vi "Teleop.vi"(10 "Match Info":T1={"Autonomous Elapsed Seconds"=0.0, "TeleOp Elapsed Seconds"=0.0, "Disabled Elapsed Seconds"=0.0, "Visited Autonomous"=FALSE, "Visited TeleOp"=FALSE, "Visited Disabled"=FALSE, "Autonomous Settings"={"Autonomous Style"=enum."Independent", "VI Refnum"=refnum}}, 11 "Call Context":T2) -> ()   [LabVIEW 2013]
doc: "This VI is called for each TeleOp packet received from the DS where the robot is not disabled. It is often used to read from the joysticks and update I/O or to update setpoints for timed control loops. It should complete and return within 20 milliseconds or it may miss DS packets."
uses:
  <vilib>/Rock Robotics/WPI/DriverStation/WPI_DriverStationDerivedRobotMode.ctl
  <vilib>/Rock Robotics/WPI/DriverStation/WPI_DriverStationMatch Info.ctl
  Robot Global Data.vi
  <vilib>/Rock Robotics/WPI/Joystick/WPI_JoystickGetSetRefNum.vi
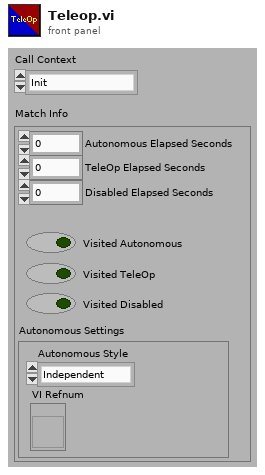
[diagram p1: front panel]
types:
  T1 = typedef "WPI_DriverStationMatch Info.ctl" = cluster{"Autonomous Elapsed Seconds":dbl, "TeleOp Elapsed Seconds":dbl, "Disabled Elapsed Seconds":dbl, "Visited Autonomous":bool, "Visited TeleOp":bool, "Visited Disabled":bool, "Autonomous Settings":cluster{"Autonomous Style":enum16{"Iterative", "Independent"}, "VI Refnum":refnum<vi>}}
  T2 = typedef "WPI_DriverStationDerivedRobotMode.ctl" = enum16{"Init", "Execute", "Stop"}
  T3 = typedef "WPI_JoystickDevRef.ctl" = cluster{"Device":T4}
  T4 = typedef "WPI_JoystickDeviceEnum.ctl" = enum16{"USB 1", "USB 2", "USB 3", "USB 4", "Kinect 1", "Kinect 2"}
  T5 = typedef "WPI_JoystickButtonState.ctl" = cluster{"Button 1":bool, "Button 2":bool, "Button 3":bool, "Button 4":bool, "Button 5":bool, "Button 6":bool, "Button 7":bool, "Button 8":bool, "Button 9":bool, "Button 10":bool, "Button 11":bool, "Button 12":bool}
  T6 = cluster{"axis 1 (x)":dbl, "axis 2 (y)":dbl, "axis 3 (throttle)":dbl, "axis 4":dbl, "axis 5":dbl, "axis 6":dbl}
  T7 = cluster{"X-Axis":dbl, "Y-Axis":dbl, "Bottom Lever":dbl, "Trigger":bool, "Button 2":bool, "Button 3":bool, "Button 4":bool, "Button 5":bool, "Button 6":bool, "Button 7":bool, "Button 8":bool, "Button 9":bool, "Button 10":bool, "Button 11":bool}
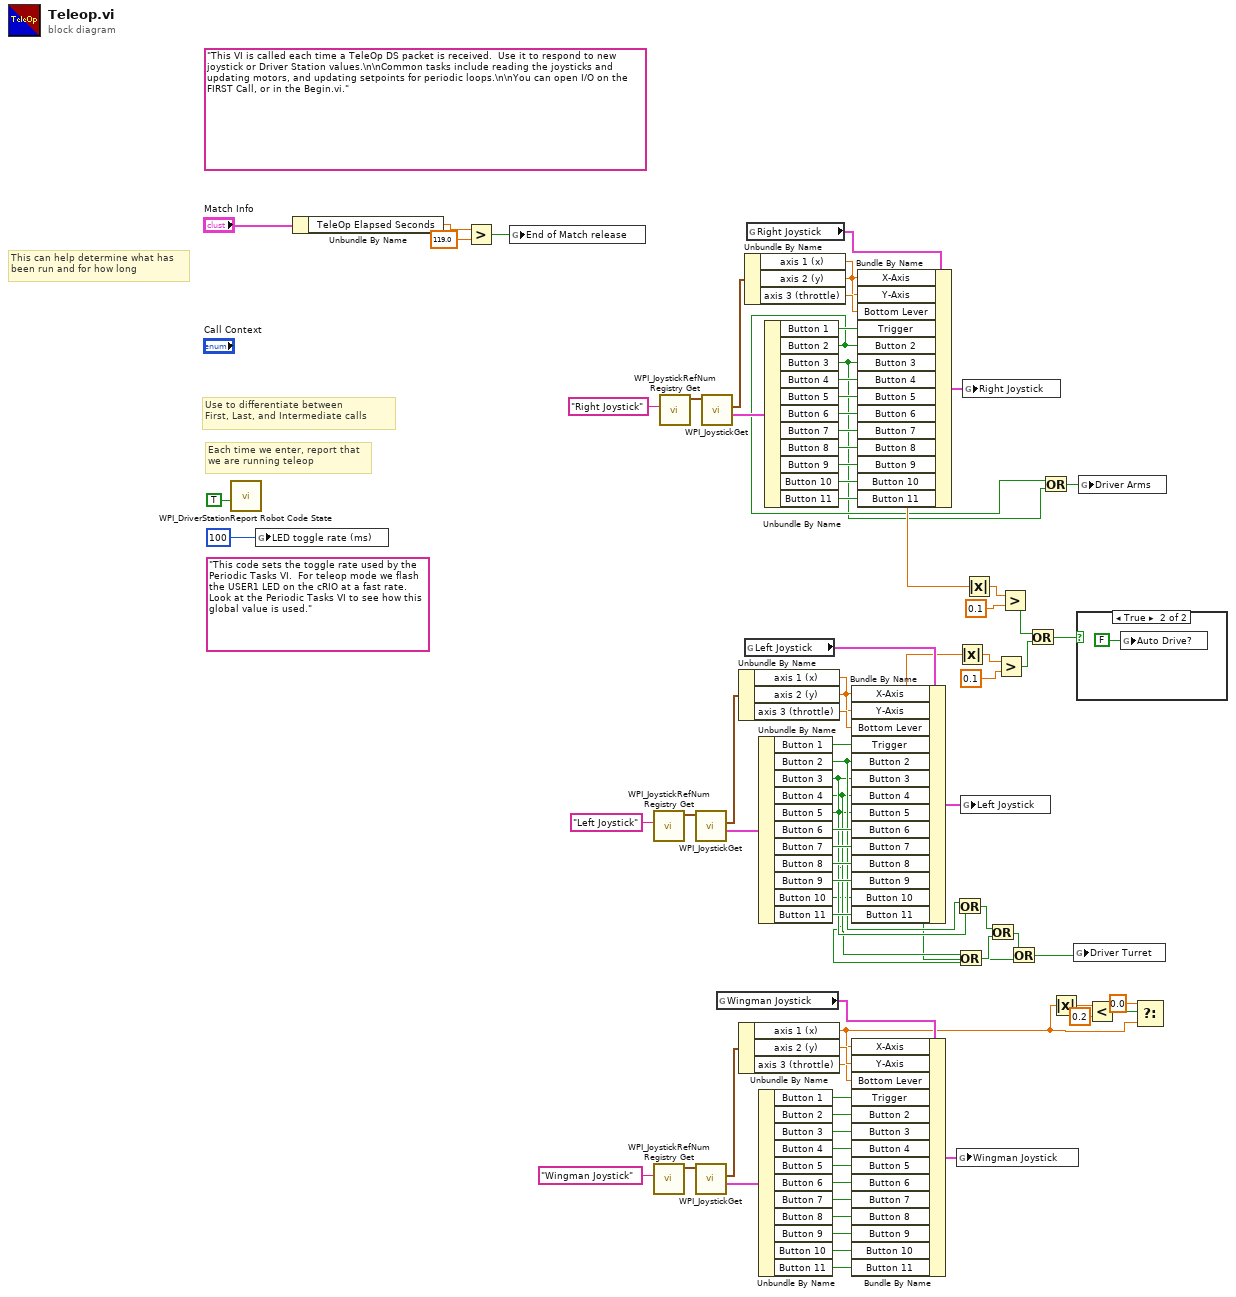
[diagram p0: block diagram]
diagram:
  (unwired) "This code sets the toggle rate used by the Periodic Tasks VI.  For teleop mode we flash the USER1 LED on the cRIO at a fast rate.  Look at the Periodic Tasks VI to see how this global value is used."
  (unwired) "This VI is called each time a TeleOp DS packet is received.  Use it to respond to new joystick or Driver Station values.\n\nCommon tasks include reading the joysticks and updating motors, and updating setpoints for periodic loops.\n\nYou can open I/O on the FIRST Call, or in the Begin.vi."
  # "Each time we enter, report that\nwe are running teleop"
  # "Use to differentiate between\nFirst, Last, and Intermediate calls"
  # "This can help determine what has\nbeen run and for how long"
  n1 = call <vilib>:"WPI_DriverStationReport Robot Code State.vi"("TeleOp"=TRUE ("Autonomous")) -> ()  [unwired: 10 in, 1 out]
  n2 = global write "Robot Global Data.vi" "LED toggle rate (ms)"(u32 100 ("LED ms toggle rate")) -> ()
  n3 = Unbundle By Name("Match Info") -> ("TeleOp Elapsed Seconds"=w39:dbl)
  n4 = Greater?(x=w39, y=119.0) -> (0:w37:bool)
  n5 = global write "Robot Global Data.vi" "End of Match release"(w37) -> ()
  n6 = call <vilib>:"WPI_JoystickRefNum Registry Get.vi"("refnum name"="Left Joystick") -> ("JoystickDevRef"=w61:T3)  [unwired: 9 in, 1 out]
  n7 = call <vilib>:"WPI_JoystickRefNum Registry Get.vi"("refnum name"="Wingman Joystick") -> ("JoystickDevRef"=w35:T3)  [unwired: 9 in, 1 out]
  n8 = call <vilib>:"WPI_JoystickRefNum Registry Get.vi"("refnum name"="Right Joystick") -> ("JoystickDevRef"=w78:T3)  [unwired: 9 in, 1 out]
  n9 = call <vilib>:"WPI_JoystickGet.vi"("JoystickDevRef"=w61) -> ("Buttons"=w59:T5, "Axes"=w60:T6)  [unwired: 4 in, 1 out]
  n10 = call <vilib>:"WPI_JoystickGet.vi"("JoystickDevRef"=w35) -> ("Buttons"=w33:T5, "Axes"=w34:T6)  [unwired: 4 in, 1 out]
  n11 = call <vilib>:"WPI_JoystickGet.vi"("JoystickDevRef"=w78) -> ("Buttons"=w76:T5, "Axes"=w77:T6)  [unwired: 4 in, 1 out]
  n12 = global read "Robot Global Data.vi" "Wingman Joystick"() -> (w32:T7)
  n13 = Unbundle By Name(w60) -> ("axis 1 (x)"=w58:dbl, "axis 2 (y)"=w48:dbl, "axis 3 (throttle)"=w57:dbl)
  n14 = Unbundle By Name(w34) -> ("axis 1 (x)"=w4:dbl, "axis 2 (y)"=w30:dbl, "axis 3 (throttle)"=w29:dbl)
  n15 = Unbundle By Name(w77) -> ("axis 1 (x)"=w73:dbl, "axis 2 (y)"=w47:dbl, "axis 3 (throttle)"=w72:dbl)
  n16 = global read "Robot Global Data.vi" "Left Joystick"() -> (w50:T7)
  n17 = global read "Robot Global Data.vi" "Right Joystick"() -> (w75:T7)
  n18 = Unbundle By Name(w59) -> ("Button 1"=w56:bool, "Button 2"=w17:bool, "Button 3"=w16:bool, "Button 4"=w15:bool, "Button 5"=w14:bool, "Button 6"=w55:bool, "Button 7"=w54:bool, "Button 8"=w53:bool, "Button 9"=w52:bool, "Button 10"=w11:bool, "Button 11"=w51:bool)
  n19 = Unbundle By Name(w33) -> ("Button 1"=w28:bool, "Button 2"=w8:bool, "Button 3"=w9:bool, "Button 4"=w27:bool, "Button 5"=w26:bool, "Button 6"=w25:bool, "Button 7"=w24:bool, "Button 8"=w23:bool, "Button 9"=w22:bool, "Button 10"=w21:bool, "Button 11"=w20:bool)
  n20 = Unbundle By Name(w76) -> ("Button 1"=w71:bool, "Button 2"=w2:bool, "Button 3"=w1:bool, "Button 4"=w70:bool, "Button 5"=w69:bool, "Button 6"=w68:bool, "Button 7"=w67:bool, "Button 8"=w66:bool, "Button 9"=w65:bool, "Button 10"=w64:bool, "Button 11"=w63:bool)
  n21 = Bundle By Name(cluster=w50, "X-Axis"=w58, "Y-Axis"=w48, "Bottom Lever"=w57, "Trigger"=w56, "Button 2"=w17, "Button 3"=w16, "Button 4"=w15, "Button 5"=w14, "Button 6"=w55, "Button 7"=w54, "Button 8"=w53, "Button 9"=w52, "Button 10"=w11, "Button 11"=w51) -> (w49:T7)
  n22 = Bundle By Name(cluster=w32, "X-Axis"=w4, "Y-Axis"=w30, "Bottom Lever"=w29, "Trigger"=w28, "Button 2"=w8, "Button 3"=w9, "Button 4"=w27, "Button 5"=w26, "Button 6"=w25, "Button 7"=w24, "Button 8"=w23, "Button 9"=w22, "Button 10"=w21, "Button 11"=w20) -> (w31:T7)
  n23 = Bundle By Name(cluster=w75, "X-Axis"=w73, "Y-Axis"=w47, "Bottom Lever"=w72, "Trigger"=w71, "Button 2"=w2, "Button 3"=w1, "Button 4"=w70, "Button 5"=w69, "Button 6"=w68, "Button 7"=w67, "Button 8"=w66, "Button 9"=w65, "Button 10"=w64, "Button 11"=w63) -> (w74:T7)
  n24 = Or(x=w17, y=w16) -> (x .or. y?=w19:bool)
  n25 = Or(x=w15, y=w14) -> (x .or. y?=w18:bool)
  n26 = Absolute Value(x=w48) -> (abs(x)=w44:dbl)
  n27 = global write "Robot Global Data.vi" "Wingman Joystick"(w31) -> ()
  n28 = global write "Robot Global Data.vi" "Left Joystick"(w49) -> ()
  n29 = global write "Robot Global Data.vi" "Right Joystick"(w74) -> ()
  n30 = Absolute Value(x=w47) -> (abs(x)=w46:dbl)
  n31 = Or(x=w19, y=w18) -> (x .or. y?=w13:bool)
  n32 = Greater?(x=w44, y=0.1) -> (0:w42:bool)
  n33 = Greater?(x=w46, y=0.1) -> (0:w41:bool)
  n34 = Or(x=w13, y=w11) -> (x .or. y?=w12:bool)
  n35 = Or(x=w41, y=w42) -> (x .or. y?=w40:bool)
  n36 = Or(x=w2, y=w1) -> (x .or. y?=w10:bool)
  n37 = Absolute Value(x=w4) -> (abs(x)=w5:dbl)
  n38 = global write "Robot Global Data.vi" "Driver Turret"(w12) -> ()
  n39 = case shown="True" w40 {
    frame False {
    }
    frame True {
      n40 = global write "Robot Global Data.vi" "Auto Drive?"(FALSE ("Auto Drive?")) -> ()
    }
  }
  n41 = global write "Robot Global Data.vi" "Driver Arms"(w10) -> ()
  n42 = Less?(x=w5, y=0.2) -> (x < y?=w6:bool)
  n43 = Select(t=0.0, s=w6, f=w4) -> ()  [unwired: 1 out]
